vi "FRCweb2iniTeamList.vi"() -> ()   [LabVIEW 2017]
uses:
  <vilib>/Utility/config.llb/Write Key (String).vi
  <vilib>/Utility/config.llb/NI_LVConfig.lvlib
panel:
  out "Select":string
  in  "Event":string(combo)
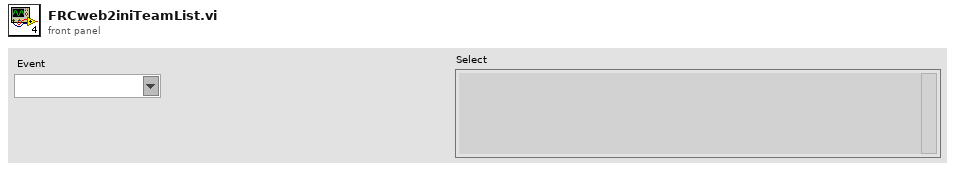
[diagram p1: front panel]
types:
  T1 = typedef "NI_LVConfig.lvlib/Config Data RefNum.ctl" = refnum<k1>
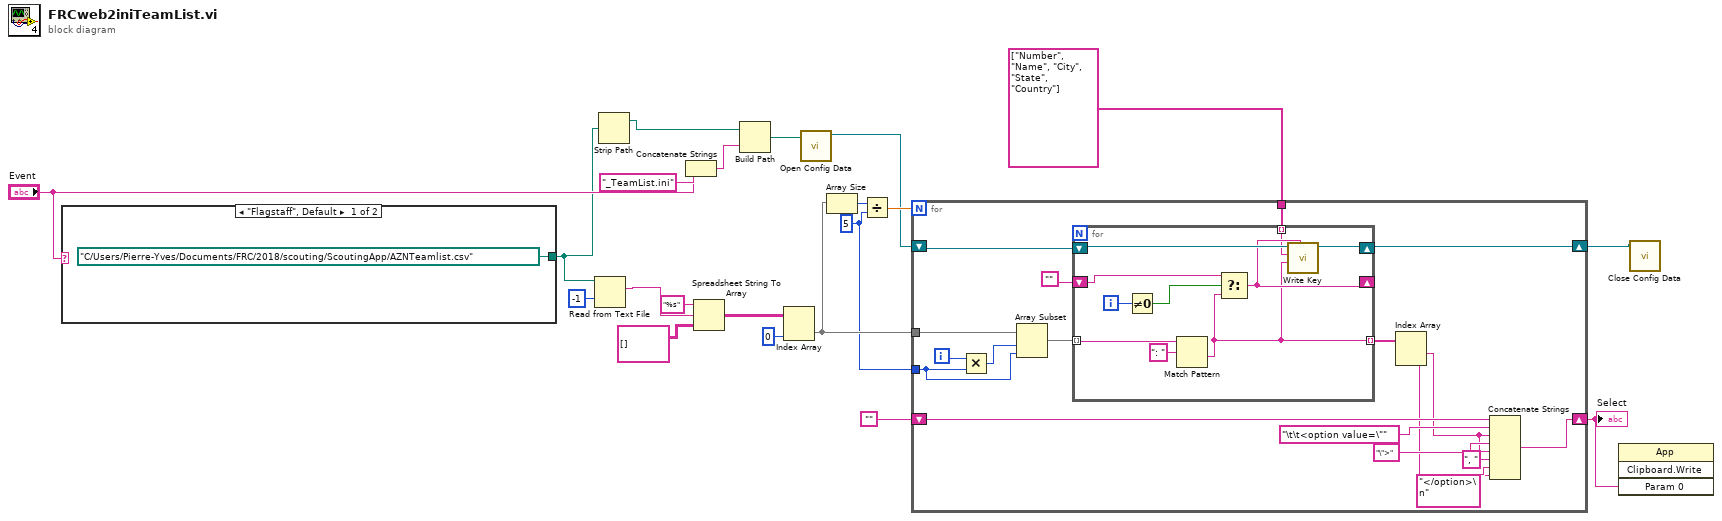
[diagram p0: block diagram]
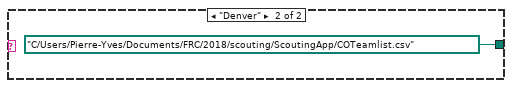
[diagram p2: hidden frame]
diagram:
  w12 = 5 ("y")
  n1 = case shown="\"Flagstaff\", Default" "Event" {
    tunnel: [path "C:/Users/Pierre-Yves/Documents/FRC/2018/scouting/ScoutingApp/AZNTeamlist.csv" ("file (use dialog)") path "C:/Users/Pierre-Yves/Documents/FRC/2018/scouting/ScoutingApp/COTeamlist.csv" ("file (use dialog)")] -> w1
    frame "Flagstaff", Default {
    }
    frame "Denver" {
    }
  }
  n2 = Read from Text File(file (use dialog)=w1, count=-1) -> (text=w18:string)  [unwired: 2 in, 3 out]
  n3 = Strip Path(path=w1) -> (stripped path=w11:path)  [unwired: 1 out]
  n4 = Concatenate Strings("Event", "_TeamList.ini" ("string")) -> (w9:string)
  n5 = Spreadsheet String To Array(format string="%s", spreadsheet string=w18, array type (2D Dbl)=string[][] []) -> (array=w19:string[][])  [unwired: 1 in]
  n6 = Build Path(base path=w11, name or relative path=w9) -> (appended path=w8:path)
  n7 = Index Array(array=w19, index (col)=0 ("disabled index (col)")) -> (element=w15:string[])  [unwired: 1 in]
  n8 = call <vilib>:"Open Config Data.vi"("configuration file path"=w8) -> ("refnum"=w7:T1)  [unwired: 8 in, 2 out]
  n9 = Array Size(array=w15) -> (size(s)=w14:i32)
  n10 = Divide(x=w14, y=w12) -> (x/y=w13:dbl)
  n11 = for {
    N: w13 -> [_]
    tunnel: w15 -> [w41]
    tunnel: w12 -> [w38]
    shift-right: [w34] -> w6
    shift-left: w7 -> [w36]
    tunnel: string[] ["Number", "Name", "City", "State", "Country"] -> [w33]
    shift-right: [w31] -> w3
    shift-left: "" -> [w32]
    i -> [w40]
    n12 = Multiply(x=w40, y=w38) -> (x*y=w39:i32)
    n13 = Array Subset(array=w41, index=w39, length=w38) -> (w37:string[])
    n14 = for {
      tunnel: w37 -> [w51] mode=indexing
      shift-right: [w45] -> _
      shift-left: "" -> [w46]
      shift-right: [w44] -> w34
      shift-left: w36 -> [w49]
      tunnel: w33 -> [w43] mode=indexing
      tunnel: [w42] -> w29 mode=indexing
      i -> [w48]
      n15 = Not Equal To 0?(x=w48) -> (x != 0?=w47:bool)
      n16 = Match Pattern(string=w51, regular expression=": ") -> (after substring=w42:string)  [unwired: 1 in, 3 out]
      n17 = Select(t=w46, s=w47, f=w42) -> (s? t:f=w45:string)
      n18 = call-poly <vilib>:"Write Key.vi"("section"=w45, "value"=w42, "key"=w43, "refnum"=w49) -> ("refnum out"=w44:T1)  [unwired: 5 in, 2 out]
    }
    n19 = Index Array(array=w29) -> (element #1=w27:string, element #2=w25:string)  [unwired: 2 in]
    n20 = Concatenate Strings(w32, "\t\t<option value=\"", w27, "\">" ("string"), w27, ", " ("string"), w25, "</option>\n" ("string")) -> (w31:string)
  }
  "Select" <- w3
  n21 = invoke class="App" method="Clipboard.Write"("Param 0"=w3) -> ()  [unwired: 3 in, 4 out]
  n22 = call <vilib>:"Close Config Data.vi"("refnum"=w6) -> ()  [unwired: 9 in, 2 out]
